vi "Initialize.vi"(8 "error in (no error)":errorcluster, 11 "Huber Settings":T1) -> (0 "error out":errorcluster, 2 "Connection Error":bool, 3 "Huber Settings":T1)   [LabVIEW 2021, in "Huber Ministat 230 TCU.lvlib"]
uses:
  Huber Ministat 230 TCU.lvlib
  Huber Settings.ctl
  <vilib>/Instr/_visa.llb/VISA Configure Serial Port (Instr).vi
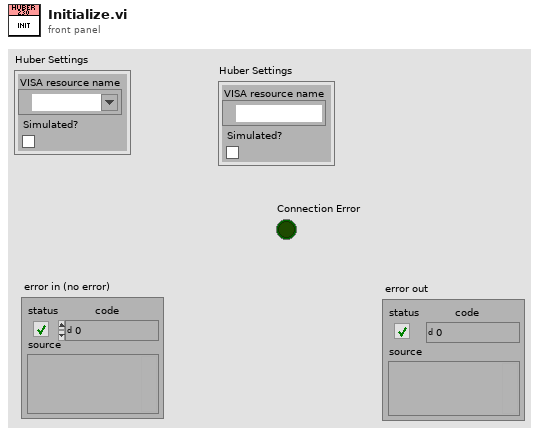
[diagram p1: front panel]
types:
  T1 = typedef "Huber Ministat 230 TCU.lvlib/Huber Settings.ctl" = cluster{"VISA resource name":refnum<visa-resource-name>, "Simulated?":bool}
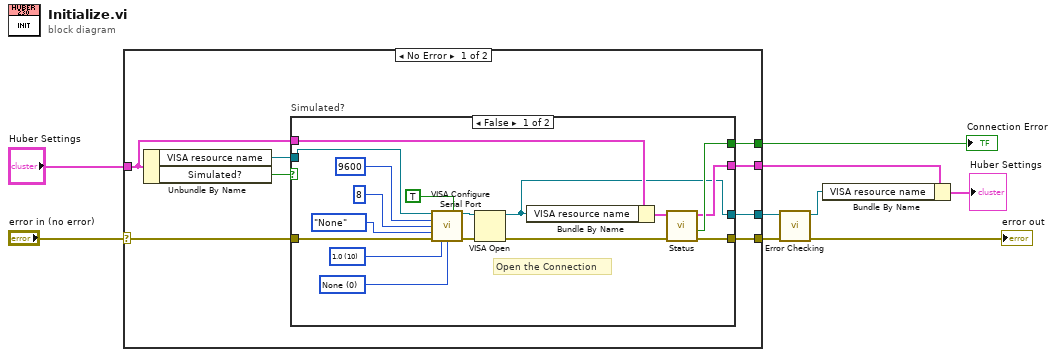
[diagram p0: block diagram]
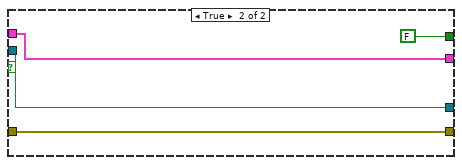
[diagram p2: hidden frame]
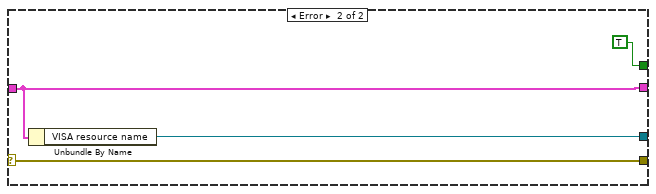
[diagram p3: hidden frame]
diagram:
  n1 = case shown="No Error" "error in (no error)" {
    selector: "error in (no error)" -> [w17 w42]
    tunnel: "Huber Settings" -> [w11 w39]
    tunnel: [w16 w42] -> w7
    tunnel: [w14 w41] -> w8
    tunnel: [w12 TRUE] -> w3
    tunnel: [w10 w39] -> w2
    frame No Error {
      n2 = Unbundle By Name(w11) -> ("VISA resource name"=w15:refnum<visa-resource-name>, "Simulated?"=w13:bool)
      n3 = case "Simulated?" shown="False" w13 {
        tunnel: w17 -> [w28 w38]
        tunnel: [w19 w38] -> w16
        tunnel: [w18 w37] -> w14
        tunnel: w15 -> [w26 w37]
        tunnel: [w21 FALSE] -> w12
        tunnel: w11 -> [w23 w35]
        tunnel: [w20 w35] -> w10
        frame False {
          w30 = u16 0 items=["None", "XON/XOFF", "RTS/CTS", "XON/XOFF & RTS/CTS", "DTR/DSR", "XON/XOFF & DTR/DSR"] ("flow control (0:none)")
          w31 = u16 10 items=["1.0"=10, "1.5"=15, "2.0"=20] ("stop bits (10: 1 bit)")
          # "Open the Connection"
          n4 = call-poly "VISA Configure Serial Port"("VISA resource name"=w26, "Enable Termination\nChar (T)"=TRUE ("Enable Termination\nChar (T)"), "baud rate (9600)"=u32 9600, "data bits (8)"=u16 8, "parity (0:none)"=enum16{"None", "Odd", "Even", "Mark", "Space"}."None", "error in (no error)"=w28, "stop bits (10: 1 bit)"=w31, "flow control (0:none)"=w30) -> ("VISA resource name out"=w27:refnum<visa-resource-name>, "error out"=w29:errorcluster)  [unwired: 6 in]
          n5 = VISA Open(error in (no error)=w29, VISA resource name=w27) -> (VISA resource name=w18:refnum<visa-resource-name>, error out=w24:errorcluster)  [unwired: 3 in]
          n6 = Bundle By Name(cluster=w23, "VISA resource name"=w18) -> (w22:T1)
          n7 = call "Status.vi"("error in (no error)"=w24, "Huber Settings In"=w22) -> ("error out"=w19:errorcluster, "Connection Error"=w21:bool, "Huber Settings Out"=w20:T1)  [unwired: 5 in, 2 out]
        }
        frame True {
        }
      }
    }
    frame Error {
      n8 = Unbundle By Name(w39) -> ("VISA resource name"=w41:refnum<visa-resource-name>)
    }
  }
  "Connection Error" <- w3
  n9 = call "Error Checking.vi"("error in (no error)"=w7, "VISA resource name"=w8) -> ("error out"=→"error out":errorcluster, "VISA resource name"=w5:refnum<visa-resource-name>)  [unwired: 7 in, 1 out]
  n10 = Bundle By Name(cluster=w2, "VISA resource name"=w5) -> (→"Huber Settings":T1)
